vi "OAT Polar Plot (Manual Label).vi"(0 "picture":picture, 1 "picture dimensions (w,h)":cluster{"width":u32, "height":u32}, 2 "polar settings":T3={"polar attributes"={"maximum"=0.0, "minimum"=0.0, "clip to min"=FALSE, "log"=FALSE, "grid color"=3381657, "plot color"=16711680, "fmt and prec"={"format"=enum."Scientific", "precision"=1}, "visible section"=8}, "desired font(Application)"=enum."Application Font", "[user-specified font]"={"Font Name:"="", "Size"=0, "Strikeout?"=FALSE, "Italic?"=FALSE, "Underline?"=FALSE, "Outline?"=FALSE, "Shadow?"=FALSE, "Bold?"=FALSE}} {"polar attributes"."minimum" format="%.2f"; "polar attributes"."maximum" format="%.2f"}, 3 "cursor attributes":T6={"layout color"=852223, "active color"=16740820, "precision"=2, "BG transparent? (T)"=TRUE, "radius"=2}, 5 "magnitude":cluster{"time/rev/rpm":dbl[], "magnitude":dbl[]} {"magnitude" format="%.2f"; "time/rev/rpm" format="%.2f"}, 7 "phase [phase lag]":cluster{"time/rev/rpm":dbl[], "phase":dbl[]} {"phase" format="%.2f"; "time/rev/rpm" format="%.2f"}, 11 "error in (no error)":errorcluster, 12 "channel settings":T2 {"probe angle [deg]" max=360 step=1; "shaft rotating direction" items=["CCW", "CW"]}, 13 "view info":T1={"dB on? (F)"=FALSE, "unwrap phase? (T)"=TRUE, "unit in degree? (T)"=TRUE}) -> (4 "new picture":picture, 10 "Cursor List [EU Position] Out":T4(array[cluster]) {"Location"."Y" format="%.2f"; "Location"."X" format="%.2f"}, 15 "error out":errorcluster)   [LabVIEW 2017]
doc: "Draws a polar plot on a picture control and adds labels. The polar plot displays the magnitude and phase of a certain order on a picture control. You must manually select the polymorphic instance to use. Use the Manual Label instance if you want to label the polar plot manually."
uses:
  <vilib>/addons/Sound and Vibration/Order Analysis/Backward Compatibility/SubVIs/OAT Polar Cursor Attributes.ctl
  <vilib>/addons/Sound and Vibration/Order Analysis/_OAT State Machine/OAT State Machine Generate Events for Booleans.vi
  <vilib>/addons/Sound and Vibration/Order Analysis/_OAT State Machine/OAT State Machine Generate Event for Numeric.vi
  <vilib>/addons/Sound and Vibration/Order Analysis/_OAT State Machine/OAT State Machine Generate Events for Numerics.vi
panel:
  in  "cursor":T5={"Name"="", "Color"=0, "Hair Style"=4, "Point Style"=2, "Name Visible"=TRUE, "Trackable"=TRUE, "Lock Style"=2, "Plot Number"=0, "Marker Index"=0, "Location"={"X"=0.5, "Y"=0.5}} {"Location"."Y" format="%.2f"; "Location"."X" format="%.2f"}
  in  "exit":bool
  in  "del cursor":bool
  in  "add cursor":bool
  out "XY Graph":cluster{"X":dbl[], "Y":dbl[]}(graph)
  out "polar plot":picture
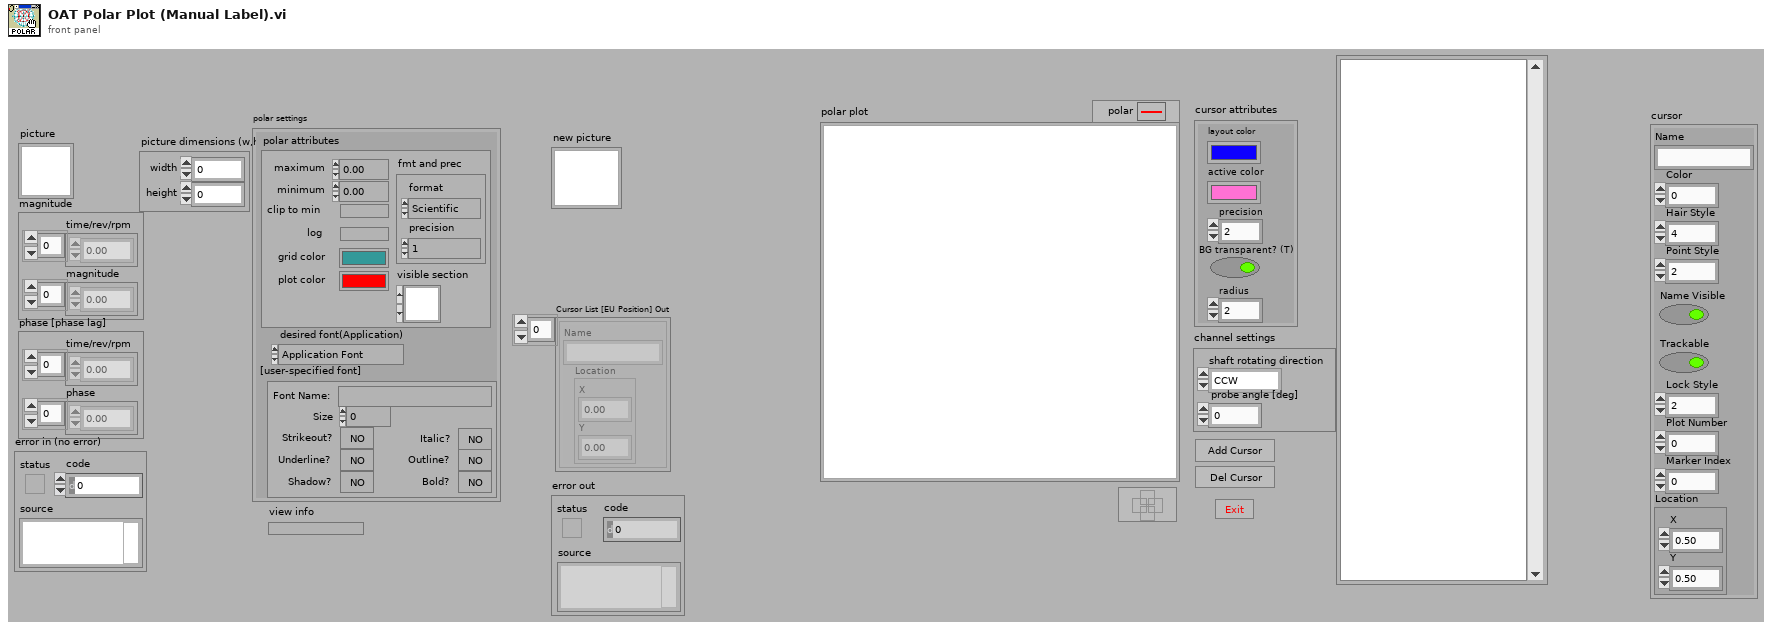
[diagram p1: front panel]
types:
  T1 = cluster{"dB on? (F)":bool, "unwrap phase? (T)":bool, "unit in degree? (T)":bool}
  T2 = cluster{"shaft rotating direction":u16, "probe angle [deg]":u16}
  T3 = cluster{"polar attributes":cluster{"maximum":dbl, "minimum":dbl, "clip to min":bool, "log":bool, "grid color":u32, "plot color":u32, "fmt and prec":cluster{"format":enum8{"Decimal", "Scientific", "Engineering", "Binary", "Octal", "Hex"}, "precision":u8}, "visible section":u16}, "desired font(Application)":enum16{"User-specified Font", "Application Font", "System Font", "Dialog Font"}, "[user-specified font]":cluster{"Font Name:":string, "Size":i16, "Strikeout?":bool, "Italic?":bool, "Underline?":bool, "Outline?":bool, "Shadow?":bool, "Bold?":bool}}
  T4 = cluster{"Name":string, "Location":cluster{"X":dbl, "Y":dbl}}[]
  T5 = cluster{"Name":string, "Color":u32, "Hair Style":u8, "Point Style":u8, "Name Visible":bool, "Trackable":bool, "Lock Style":u32, "Plot Number":u32, "Marker Index":i32, "Location":cluster{"X":dbl, "Y":dbl}}
  T6 = typedef "OAT Polar Cursor Attributes.ctl" = cluster{"layout color":u32, "active color":u32, "precision":i16, "BG transparent? (T)":bool, "radius":i16}
  T7 = cluster{"Name":string, "Color":u32, "Hair Style":u8, "Point Style":u8, "Name Visible":bool, "Trackable":bool, "Lock Style":u32, "Plot Number":u32, "Marker Index":i32, "Location":cluster{"X":dbl, "Y":dbl}}[]
  T8 = cluster{"pixel center":cluster{"x":i16, "y":i16}, "scale factors":cluster{"a":dbl, "b":dbl, "log?":bool}, "grid color":u32, "start angle":dbl, "end angle":dbl, "tick length":i16, "pixel radius":i32}
  T9 = typedef "LVBoundsTypeDef.ctl" = cluster{"Width":u32, "Height":u32}
  T10 = cluster{"Name":string, "Color":u32, "Style":u8, "Point Style":u8, "Name Visible":bool, "Allow Drag":bool, "Lock Style":u32, "Plot":u32, "Index":i32, "Position":cluster{"X":dbl, "Y":dbl}}[]
  T11 = cluster{"Name":string, "Color":u32, "Style":u8, "Point Style":u8, "Name Visible":bool, "Allow Drag":bool, "Lock Style":u32, "Plot":u32, "Index":i32, "Position":cluster{"X":dbl, "Y":dbl}}
  T12 = cluster{"Name":string, "Location":cluster{"mag":dbl, "phase":dbl}}[]
  T13 = cluster{"maximum":dbl, "minimum":dbl, "clip to min":bool, "log":bool, "grid color":u32, "plot color":u32, "fmt and prec":cluster{"format":enum8{"Decimal", "Scientific", "Engineering", "Binary", "Octal", "Hex"}, "precision":u8}, "visible section":u16}
  T14 = cluster{"polar settings":cluster{"polar attributes":cluster{"maximum":dbl, "minimum":dbl, "clip to min":bool, "log":bool, "grid color":u32, "plot color":u32, "fmt and prec":cluster{"format":enum8{"Decimal", "Scientific", "Engineering", "Binary", "Octal", "Hex"}, "precision":u8}, "visible section":u16}, "desired font(Application)":enum16{"User-specified Font", "Application Font", "System Font", "Dialog Font"}, "[user-specified font]":cluster{"Font Name:":string, "Size":i16, "Strikeout?":bool, "Italic?":bool, "Underline?":bool, "Outline?":bool, "Shadow?":bool, "Bold?":bool}}, "Draw Area Size":T9, "grid measurements out":cluster{"pixel center":cluster{"x":i16, "y":i16}, "scale factors":cluster{"a":dbl, "b":dbl, "log?":bool}, "grid color":u32, "start angle":dbl, "end angle":dbl, "tick length":i16, "pixel radius":i32}}
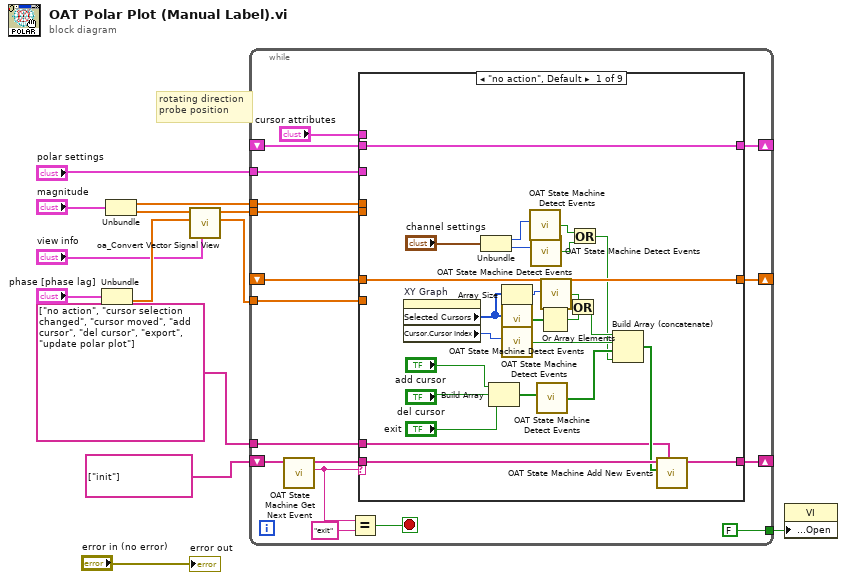
[diagram p0: block diagram]
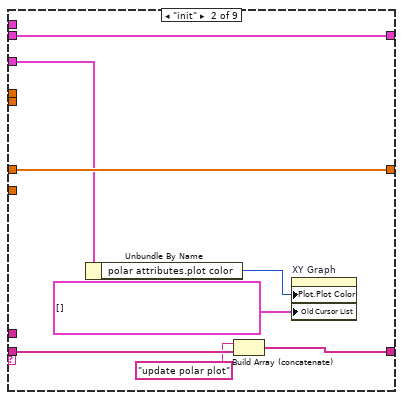
[diagram p2: hidden frame]
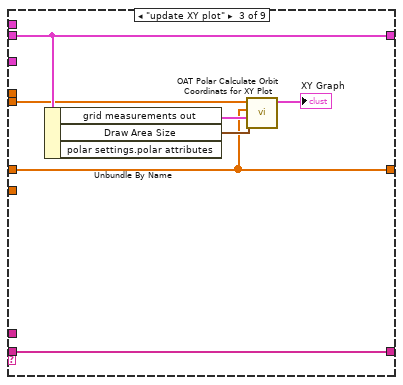
[diagram p3: hidden frame]
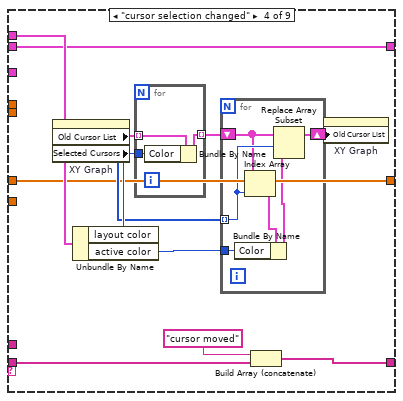
[diagram p4: hidden frame]
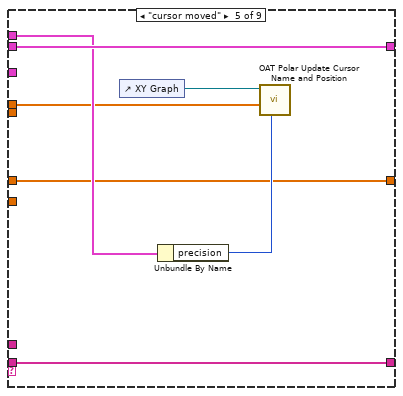
[diagram p5: hidden frame]
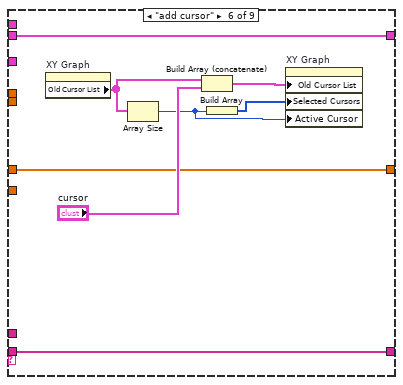
[diagram p6: hidden frame]
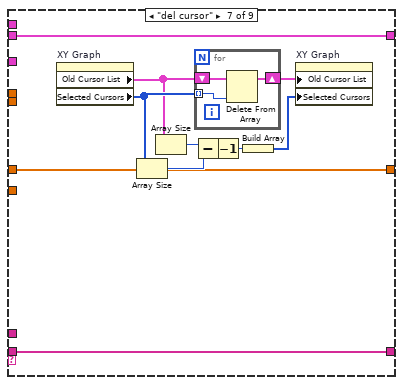
[diagram p7: hidden frame]
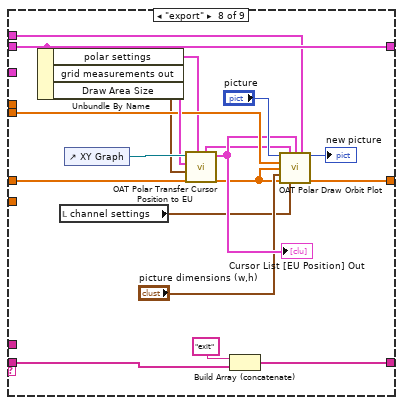
[diagram p8: hidden frame]
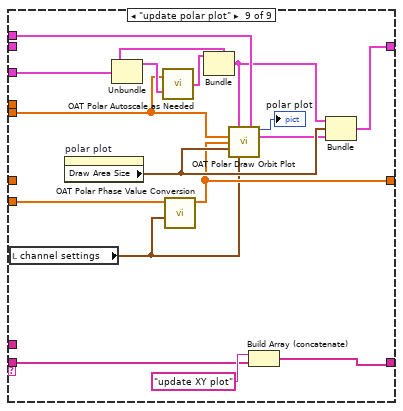
[diagram p9: hidden frame]
diagram:
  # "rotating direction\nprobe position"
  n1 = Unbundle("phase [phase lag]") -> ("phase"=w4:dbl[])  [unwired: 1 out]
  n2 = Unbundle("magnitude") -> ("time/rev/rpm"=w7:dbl[], "magnitude"=w5:dbl[])
  n3 = call <vilib>:"oa_Convert Vector Signal View.vi"("view"="view info", "phase"=w4, "magnitude"=w5) -> ("phase out"=w1:dbl[], "magnitude out"=w3:dbl[])  [unwired: 7 in]
  n4 = while {
    shift-left: _ -> [w22]
    shift-right: [w23] -> _
    tunnel: string[] ["no action", "cursor selection changed", "cursor moved", "add cursor", "del cursor", "export", "update polar plot"] ("Event Queue Out") -> [w24]
    shift-left: string[] ["init"] ("Event Queue Out") -> [w30]
    shift-right: [w28] -> _
    tunnel: w3 -> [w20]
    tunnel: w7 -> [w19]
    tunnel: [FALSE] -> w6
    shift-right: [w16] -> _
    shift-left: _ -> [w17]
    tunnel: w1 -> [w15]
    tunnel: "polar settings" -> [w14]
    stop <- w25 stop-if-true
    n5 = call <vilib>:"OAT State Machine Get Next Event.vi"("event queue in"=w30) -> ("next event"=w27:string, "event queue out"=w29:string[])  [unwired: 5 in]
    n6 = Equal?(x=w27, y="exit") -> (x = y?=w25:bool)
    n7 = case shown="\"no action\", Default" w27 {
      tunnel: w29 -> [w55 w63 w70 w78 w98 w105 w117 w136 w146]
      tunnel: [w54 w61 w70 w77 w98 w105 w117 w135 w145] -> w28
      tunnel: w24 -> [w50 _ _ _ _ _ _ _ _]
      tunnel: "cursor attributes" -> [_ _ _ w81 w95 _ _ w129 w151]
      tunnel: [w45 w59 w69 w72 w96 w103 w108 w134 w148] -> w23
      tunnel: w22 -> [w45 w59 w69 w72 w96 w103 w108 w134 _]
      tunnel: w20 -> [_ _ w66 _ _ _ _ w128 w139]
      tunnel: w19 -> [_ _ _ _ w93 _ _ _ _]
      tunnel: w17 -> [w37 w58 w64 w71 w92 w100 w107 w123 _]
      tunnel: [w37 w58 w64 w71 w92 w100 w107 w123 w140] -> w16
      tunnel: w15 -> [_ _ _ _ _ _ _ _ w141]
      tunnel: w14 -> [_ w56 _ _ _ _ _ _ w143]
      frame "no action", Default {
        n8 = property on="XY Graph" class="XYGraph (strict)"() -> ("Selected Cursors"=w49:u32[], "Cursor.Cursor Index"=w39:i32)  [unwired: 2 in, 2 out]
        n9 = Unbundle("channel settings") -> ("shaft rotating direction"=w32:u16, "probe angle [deg]"=w31:u16)
        n10 = Build Array("add cursor", "del cursor", "exit") -> (w41:bool[])
        n11 = Array Size(array=w49) -> (size(s)=w40:i32)
        n12 = call-poly <vilib>:"OAT State Machine Detect Events.vi"("Numerics"=w49) -> ("Event Found?"=w53:bool[])  [unwired: 7 in]
        n13 = call-poly <vilib>:"OAT State Machine Detect Events.vi"("Numeric"=w39) -> ("Event"=w38:bool)  [unwired: 7 in]
        n14 = call-poly <vilib>:"OAT State Machine Detect Events.vi"("Numeric"=w32) -> ("Event"=w36:bool)  [unwired: 7 in]
        n15 = call-poly <vilib>:"OAT State Machine Detect Events.vi"("Numeric"=w31) -> ("Event"=w35:bool)  [unwired: 7 in]
        n16 = call-poly <vilib>:"OAT State Machine Detect Events.vi"("Booleans"=w41) -> ("Event Found?"=w52:bool[])  [unwired: 7 in]
        n17 = Or Array Elements(Boolean array=w53) -> (logical OR=w47:bool)
        n18 = call-poly <vilib>:"OAT State Machine Detect Events.vi"("Numeric"=w40) -> ("Event"=w48:bool)  [unwired: 7 in]
        n19 = Or(x=w48, y=w47) -> (x .or. y?=w46:bool)
        n20 = Or(x=w36, y=w35) -> (x .or. y?=w34:bool)
        n21 = Build Array (concatenate)(w46, w38, w52, w34) -> (w51:bool[])
        n22 = call <vilib>:"OAT State Machine Add New Events.vi"("Event Names"=w50, "New Events"=w51, "Event Queue In"=w55) -> ("Event Queue Out"=w54:string[])  [unwired: 8 in]
      }
      frame "init" {
        n23 = Unbundle By Name(w56) -> ("polar attributes.plot color"=w57:u32)
        n24 = Build Array (concatenate)("update polar plot", w63) -> (w61:string[])
        n25 = property on="XY Graph" class="XYGraph (strict)"("Plot.Plot Color"=w57, "Old Cursor List"=T7 [] ("Cursor List")) -> ()  [unwired: 2 in, 2 out]
      }
      frame "update XY plot" {
        n26 = Unbundle By Name(w69) -> ("grid measurements out"=w68:T8, "Draw Area Size"=w67:T9)  [unwired: 1 out]
        n27 = call <vilib>:"OAT Polar Calculate Orbit Coordinats for XY Plot.vi"("picture dimensions (w,h)"=w67, "grid measurements"=w68, "phases"=w64, "magnitudes"=w66) -> ("orbit for XY plot"=→"XY Graph":cluster{"X":dbl[], "Y":dbl[]})  [unwired: 7 in]
      }
      frame "cursor selection changed" {
        n28 = property on="XY Graph" class="XYGraph (strict)"() -> ("Old Cursor List"=w82:T10, "Selected Cursors"=w79:u32[])  [unwired: 2 in, 2 out]
        n29 = Unbundle By Name(w81) -> ("layout color"=w80:u32, "active color"=w74:u32)
        n30 = for {
          tunnel: w82 -> [w91] mode=indexing
          tunnel: w80 -> [w90]
          tunnel: [w89] -> w75 mode=indexing
          n31 = Bundle By Name(cluster=w91, "Color"=w90) -> (w89:T11)
        }
        n32 = for {
          tunnel: w79 -> [w88] mode=indexing
          shift-right: [w86] -> w73
          shift-left: w75 -> [w87]
          tunnel: w74 -> [w85]
          n33 = Index Array(array=w87, index=w88) -> (element=w84:T11)
          n34 = Bundle By Name(cluster=w84, "Color"=w85) -> (w83:T11)
          n35 = Replace Array Subset(array=w87, new element=w83, index=w88) -> (w86:T10)
        }
        n36 = Build Array (concatenate)("cursor moved", w78) -> (w77:string[])
        n37 = property on="XY Graph" class="XYGraph (strict)"("Old Cursor List"=w73) -> ()  [unwired: 2 in, 2 out]
      }
      frame "cursor moved" {
        n38 = control-ref of="XY Graph"() -> (w97:refnum<vi>)
        n39 = Unbundle By Name(w95) -> ("precision"=w94:i16)
        n40 = call <vilib>:"OAT Polar Update Cursor Name and Position.vi"("precision (2)"=w94, "X"=w93, "XY Graph"=w97) -> ()  [unwired: 8 in, 1 out]
      }
      frame "add cursor" {
        n41 = property on="XY Graph" class="XYGraph (strict)"() -> ("Old Cursor List"=w99:T10)  [unwired: 2 in, 2 out]
        n42 = Array Size(array=w99) -> (size(s)=w101:i32)
        n43 = Build Array (concatenate)(w99, "cursor") -> (w106:T7)
        n44 = Build Array(w101) -> (w102:i32[])
        n45 = property on="XY Graph" class="XYGraph (strict)"("Old Cursor List"=w106, "Selected Cursors"=w102, "Active Cursor"=w101) -> ()  [unwired: 2 in, 2 out]
      }
      frame "del cursor" {
        n46 = property on="XY Graph" class="XYGraph (strict)"() -> ("Old Cursor List"=w113:T10, "Selected Cursors"=w116:u32[])  [unwired: 2 in, 2 out]
        n47 = Array Size(array=w116) -> (size(s)=w114:i32)
        n48 = Array Size(array=w113) -> (size(s)=w115:i32)
        n49 = Subtract(x=w115, y=w114) -> (x-y=w111:i32)
        n50 = for {
          tunnel: w116 -> [w120] mode=indexing
          shift-right: [w118] -> w112
          shift-left: w113 -> [w119]
          n51 = Delete From Array(array=w119, index=w120) -> (array with subset deleted=w118:T10)  [unwired: 1 in, 1 out]
        }
        n52 = Decrement(x=w111) -> (x-1=w109:i32)
        n53 = Build Array(w109) -> (w110:i32[])
        n54 = property on="XY Graph" class="XYGraph (strict)"("Old Cursor List"=w112, "Selected Cursors"=w110) -> ()  [unwired: 2 in, 2 out]
      }
      frame "export" {
        n55 = Unbundle By Name(w134) -> ("polar settings"=w122:T3, "grid measurements out"=w130:T8, "Draw Area Size"=w127:T9)
        n56 = local read "channel settings"() -> (w121:T2)
        n57 = control-ref of="XY Graph"() -> (w131:refnum<vi>)
        n58 = call <vilib>:"OAT Polar Transfer Cursor Position to EU.vi"("polar settings"=w122, "picture \ndimensions (w,h)"=w127, "grid measurements"=w130, "XY Graph"=w131) -> ("Cursor List (EU position]"=w126:T12, "polar settings out"=w124:T3)  [unwired: 6 in]
        "Cursor List [EU Position] Out" <- w126
        n59 = Build Array (concatenate)("exit", w136) -> (w135:string[])
        n60 = call <vilib>:"OAT Polar Draw Orbit Plot.vi"("picture"="picture", "polar settings"=w124, "Cursor List (EU position]"=w126, "cursor attributes"=w129, "magnitudes (even angular)"=w128, "phases"=w123, "picture \ndimensions (w,h)"="picture dimensions (w,h)", "channel settings"=w121) -> ("picture out"=→"new picture":picture)  [unwired: 6 in, 1 out]
      }
      frame "update polar plot" {
        n61 = local read "channel settings"() -> (w138:T2)
        n62 = property on="polar plot" class="Pict"() -> ("Draw Area Size"=w153:T9)  [unwired: 2 in, 2 out]
        n63 = Unbundle(w143) -> ("polar attributes"=w150:T13)  [unwired: 2 out]
        n64 = call <vilib>:"OAT Polar Autoscale as Needed.vi"("polar attributes"=w150, "magnitudes (even angular)"=w139) -> ("polar attributes"=w149:T13)
        n65 = call <vilib>:"OAT Polar Phase Value Conversion.vi"("channel settings"=w138, "phases in"=w141) -> ("phases out"=w140:dbl[])  [unwired: 9 in]
        n66 = Bundle(cluster=w143, "polar attributes"=w149) -> (w142:T3)  [unwired: 2 in]
        n67 = call <vilib>:"OAT Polar Draw Orbit Plot.vi"("polar settings"=w142, "cursor attributes"=w151, "magnitudes (even angular)"=w139, "phases"=w140, "picture \ndimensions (w,h)"=w153, "channel settings"=w138) -> ("picture out"=→"polar plot":picture, "grid measurements out"=w152:T8)  [unwired: 8 in]
        n68 = Build Array (concatenate)("update XY plot", w146) -> (w145:string[])
        n69 = Bundle("polar settings"=w142, "Draw Area Size"=w153, "grid measurements out"=w152) -> (w148:T14)  [unwired: 1 in]
      }
    }
  }
  n70 = property class="VI"("Front Panel Window:Open"=w6) -> ()  [unwired: 2 in, 2 out]
  "error out" <- "error in (no error)"
